vi "Controller - FGV Timer.vi"(7 "CMD Timer":T1, 8 "error in (no error)":errorcluster, 11 "Target Time":dbl) -> (0 "error out":errorcluster, 2 "Elapsed?":bool, 3 "Elapsed Time":dbl)   [LabVIEW 2017]
doc: "Pausable Timer based on Functional Global Variable"
uses:
  Controls/Elevator CMD Timer.ctl
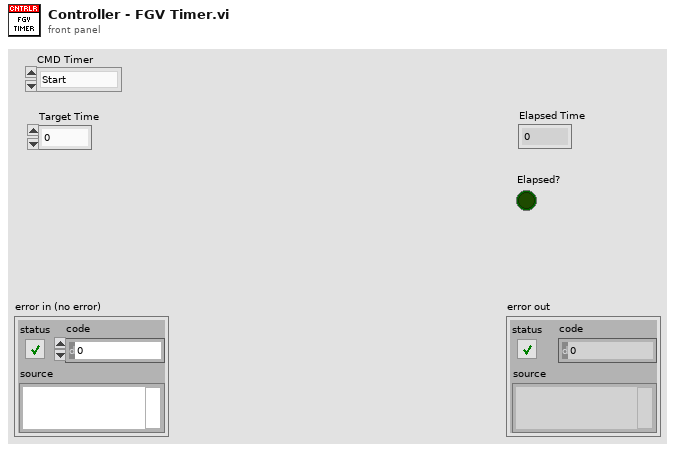
[diagram p1: front panel]
types:
  T1 = typedef "Elevator CMD Timer.ctl" = enum16{"Start", "Get Time", "Pause", "Unpause"}
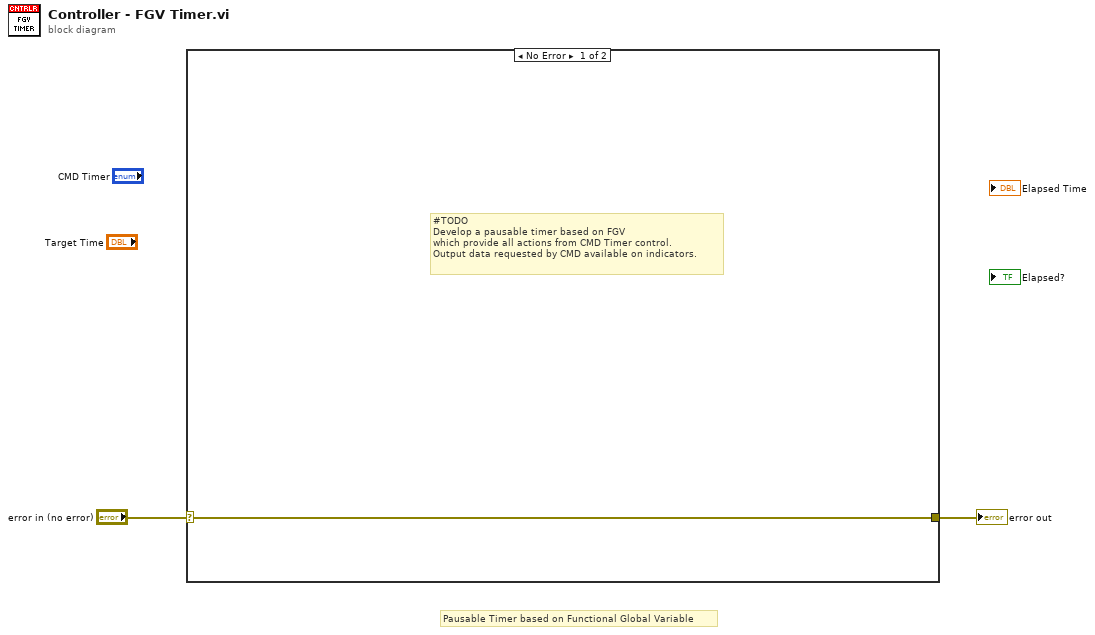
[diagram p0: block diagram]
diagram:
  # "Pausable Timer based on Functional Global Variable"
  n1 = case shown="No Error" "error in (no error)" {
    selector: "error in (no error)" -> [w3 w4]
    tunnel: [w3 w4] -> w1
    frame No Error {
      # "#TODO\nDevelop a pausable timer based on FGV\nwhich provide all actions from CMD Timer control.\nOutput data requested by CMD available on indicators."
    }
    frame Error {
    }
  }
  "error out" <- w1
